vi "SW_Select_User_v.2.vi"() -> ()   [LabVIEW 2016]
uses:
  <vilib>/Utility/miscctls.llb/LVPointTypeDef.ctl
  <vilib>/Utility/config.llb/NI_LVConfig.lvlib
panel:
  out "TestComm indicator for Latching inside Events workaround":bool
  in  "Login tab":enum32{"Login", "Settings", "Manage users"}(tab)
  in  "Go to Tracker":bool
  in  "Select User":u16(ring) items=["Admin"]
  in  "Enter password":string
  in  "Jump to tracking":bool
  out "Comm. test results":bool
  in  "Test VISA Comms":bool
  in  "Save Settings":bool
  in  "VISA":refnum<visa-resource-name>="Tracker"
  in  "Cancel Users Update":bool
  in  "Save Users":bool
  in  "... or add new one":string
  in  "Reset or create password":string
  in  "Select User for update":u16(ring) items=["Researcher"]
  in  "Delete current user":bool
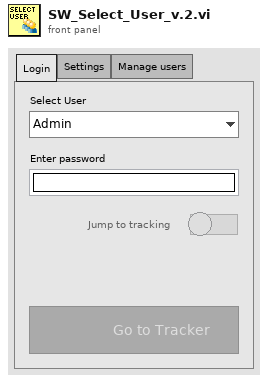
[diagram p1: front panel]
types:
  T1 = cluster{"Numeric Control":u32, "Numeric Control":u32}[]
  T2 = typedef "LVPointTypeDef.ctl" = cluster{"Horizontal":i16, "Vertical":i16}
  T3 = cluster{"Tabs":refnum<vi>, "Select User at login page":refnum<vi>, "Enter password":refnum<vi>, "Jump to tracking":refnum<vi>, "Test VISA Comms button":refnum<vi>, "Comm. test results indicator":refnum<vi>}
  T4 = typedef "NI_LVConfig.lvlib/Config Data RefNum.ctl" = refnum<k1>
  T5 = typedef "eventvkey.ctl" = enum16{"ASCII", "Enter", "Return", "Shift", "Ctrl", "Alt", "Cmd", "Opt", "Caps", "NumLock", "Clear", "Break", "Up", "Down", "Left", "Right", "Insert", "Delete", "Home", "End", "PageUp", "PageDown", "Escape", "Help", "Pause", "ScrollLock", "F1", "F2", "F3", "F4", "F5", "F6", "F7", "F8", "F9", "F10", "F11", "F12", "F13", "F14", "F15", "F16", "F17", "F18", "F19", "F20", "F21", "F22", "F23", "F24", "Play", "VolumeUp", "VolumeDown", "Mute", "Two Byte Char"}
  T6 = enum32{"Page Enabled", "Page Disabled", "Page Disabled & Grayed"}
  T7 = enum8{"Enabled", "Disabled", "Disabled and Grayed Out"}
  T8 = cluster{"Data acquisition status":refnum<notifier>, "Play/Pause status":refnum<notifier>, "Recording status":refnum<notifier>}
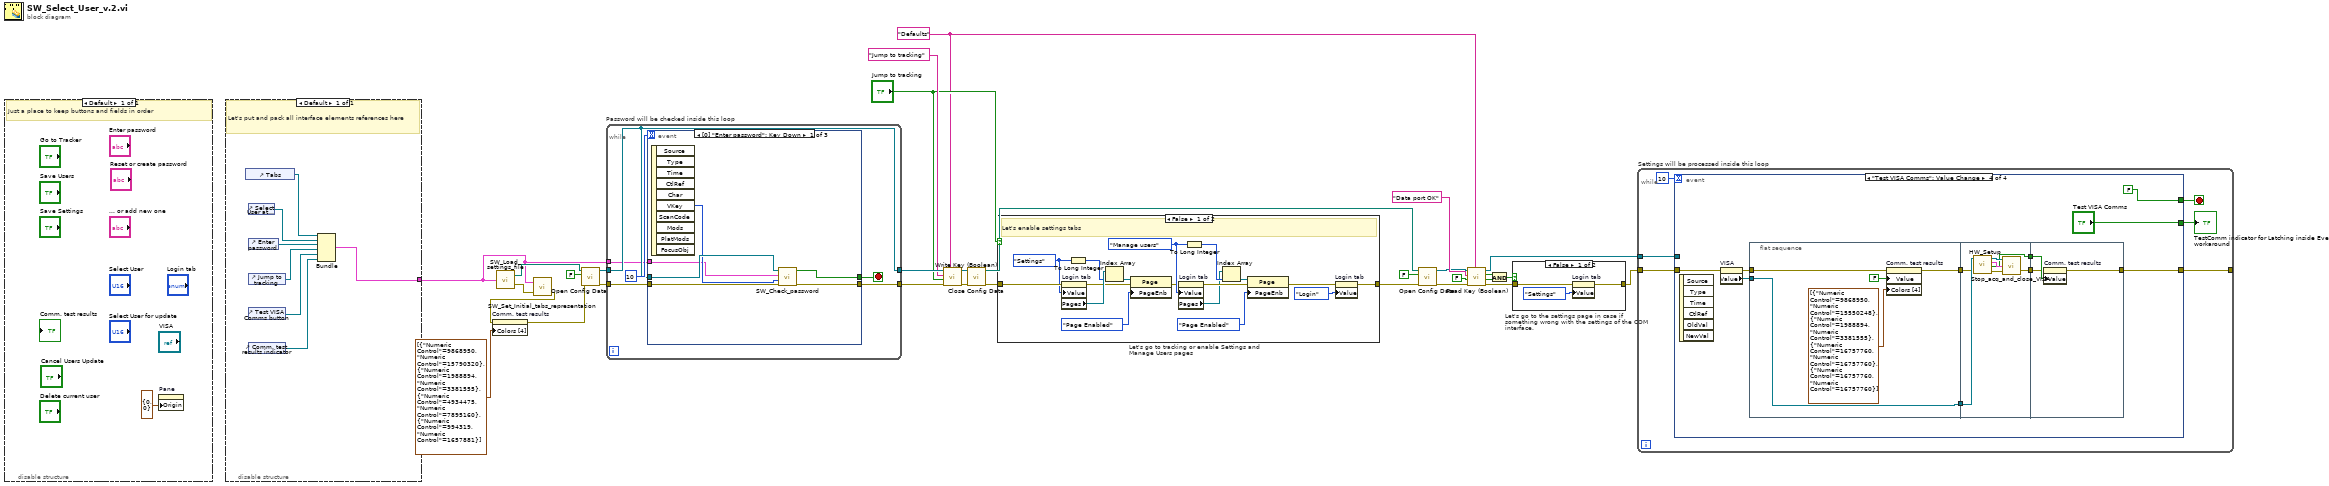
[diagram p0: block diagram]
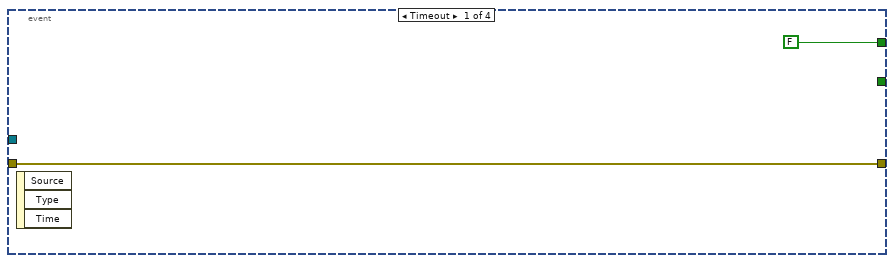
[diagram p2: hidden frame]
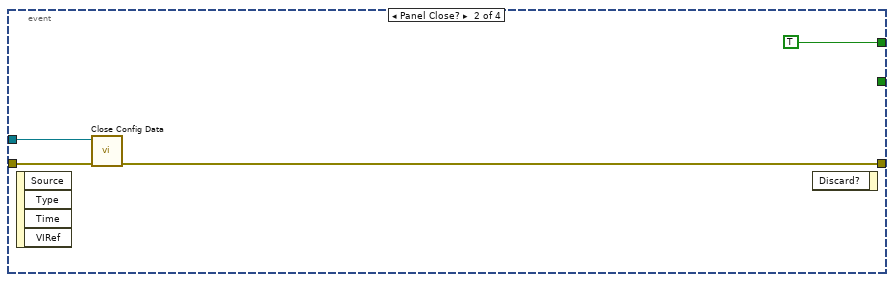
[diagram p3: hidden frame]
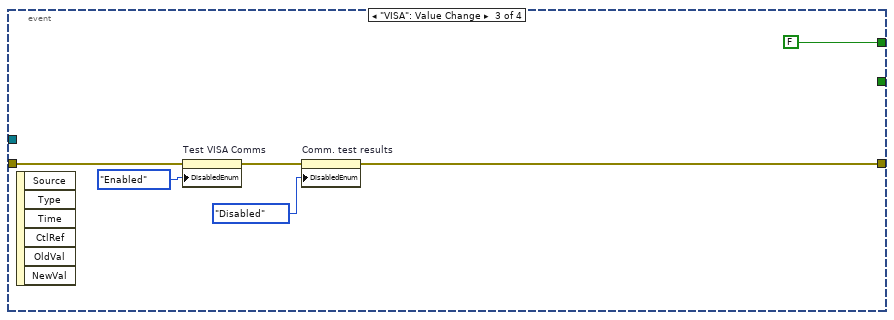
[diagram p4: hidden frame]
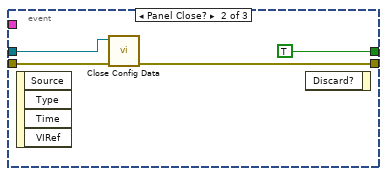
[diagram p7: hidden frame]
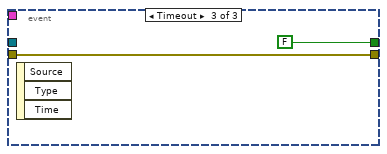
[diagram p8: hidden frame]
diagram:
  w22 = "Defaults" ("section")
  n1 = disable-structure shown="Default" {
    frame Enabled {
      # "Just a place to keep buttons and fields in order"
      n2 = property on="Pane" class="Pane"("Origin"=T2 {"Horizontal"=0, "Vertical"=0}) -> ()  [unwired: 2 in, 2 out]
    }
  }
  n3 = disable-structure "Conditional Disable Structure" shown="Default" {
    disable-tunnel: [w32] -> w1
    frame Enabled {
      # "Let's put and pack all interface elements references here"
      n4 = control-ref of="Tabs"() -> (w38:refnum<vi>)
      n5 = control-ref of="Select User at login page"() -> (w37:refnum<vi>)
      n6 = control-ref of="Enter password"() -> (w36:refnum<vi>)
      n7 = control-ref of="Jump to tracking"() -> (w35:refnum<vi>)
      n8 = control-ref of="Test VISA Comms button"() -> (w34:refnum<vi>)
      n9 = control-ref of="Comm. test results indicator"() -> (w33:refnum<vi>)
      n10 = Bundle("Tabs"=w38, "Select User at login page"=w37, "Enter password"=w36, "Jump to tracking"=w35, "Test VISA Comms button"=w34, "Comm. test results indicator"=w33) -> (w32:T3)  [unwired: 1 in]
    }
  }
  n11 = call "SW_Load_settings_file.vi"("Controls references"=w1) -> ("Config file path"=w7:path, "error out"=w28:errorcluster)
  n12 = call "SW_Set_Initial_tabs_representation.vi"("error in (no error)"=w28, "Controls references"=w1) -> ("error out"=w3:errorcluster)  [unwired: 1 in]
  n13 = property on="Comm. test results" class="Bool (strict)"(error in=w3, "Colors [4]"=T1 [{"Numeric Control"=9868950, "Numeric Control"=15790320}, {"Numeric Control"=1988894, "Numeric Control"=3381555}, {"Numeric Control"=4934475, "Numeric Control"=7895160}, {"Numeric Control"=994319, "Numeric Control"=1657881}]) -> (error out=w4:errorcluster)  [unwired: 1 in, 1 out]
  n14 = call <vilib>:"Open Config Data.vi"("error in (no error)"=w4, "create file if necessary (T)"=FALSE, "configuration file path"=w7) -> ("error out"=w29:errorcluster, "refnum"=w30:T4)  [unwired: 6 in, 1 out]
  n15 = while "Password will be checked inside this loop" {
    tunnel: w29 -> [w43]
    tunnel: w30 -> [w41]
    tunnel: [w42] -> w26
    tunnel: [w41] -> w27
    tunnel: w1 -> [w39]
    stop <- w40 stop-if-true
    n16 = event shown="[0] \"Enter password\": Key Down" {
      selector: _ -> [_ _ _]
      dyn-events: _ -> [_ _ _]
      timeout: 10 -> [_ _ _]
      tunnel: w43 -> [w50 w53 w55]
      tunnel: w41 -> [w49 w51 _]
      tunnel: [w47 TRUE ("Stop the loop") FALSE] -> w40
      tunnel: [w46 w52 w55] -> w42
      tunnel: w39 -> [w45 _ _]
      event "Enter password": Key Down {
        n17 = event-data() -> ("VKey"=w48:T5)  [unwired: 1 in, 9 out]
        n18 = call "SW_Check_password.vi"("error in (no error)"=w50, "Entered key"=w48, "Controls references"=w45, "Configuration file refnum in"=w49) -> ("error out"=w46:errorcluster, "Stop the loop"=w47:bool)  [unwired: 6 in]
      }
      event Panel Close? {
        n19 = event-data() -> ()  [unwired: 1 in, 4 out]
        n20 = call <vilib>:"Close Config Data.vi"("error in (no error)"=w53, "refnum"=w51) -> ("error out"=w52:errorcluster)  [unwired: 8 in, 1 out]
        n21 = event-data() -> ()  [unwired: 2 in, 1 out]
      }
      event Timeout {
        n22 = event-data() -> ()  [unwired: 1 in, 3 out]
      }
    }
  }
  n23 = call <vilib>:"Write Key (Boolean).vi"("section"=w22, "error in (no error)"=w26, "value"="Jump to tracking", "key"="Jump to tracking", "refnum"=w27) -> ("error out"=w16:errorcluster, "refnum out"=w14:T4)  [unwired: 4 in, 1 out]
  n24 = call <vilib>:"Close Config Data.vi"("error in (no error)"=w16, "refnum"=w14) -> ("error out"=w15:errorcluster, "file path"=w13:path)  [unwired: 8 in]
  n25 = case "Let's go to tracking or enable Settings and Manage Users pages" shown="False" "Jump to tracking" {
    tunnel: w15 -> [w73 w74]
    tunnel: [w58 w74] -> w12
    frame False {
      w62 = enum32{"Login", "Settings", "Manage users"}."Manage users" ("Login tab")
      w71 = enum32{"Login", "Settings", "Manage users"}."Settings" ("Login tab")
      # "Let's enable settings tabs"
      n26 = property on="Login tab" class="TabCtl (strict)"(error in=w73, "Value"=w71) -> (error out=w68:errorcluster, "Pages"=w72:refnum<vi>[])  [unwired: 1 in, 1 out]
      n27 = To Long Integer(number=w71) -> (32bit integer=w70:i32)
      n28 = Index Array(array=w72, index=w70) -> (element=w69:refnum<vi>)
      n29 = property class="Page"(reference=w69, error in=w68, "PageEnb"=T6."Page Enabled" ("Page Enabled State")) -> (error out=w60:errorcluster)  [unwired: 1 out]
      n30 = property on="Login tab" class="TabCtl (strict)"(error in=w60, "Value"=w62) -> (error out=w65:errorcluster, "Pages"=w61:refnum<vi>[])  [unwired: 1 in, 1 out]
      n31 = To Long Integer(number=w62) -> (32bit integer=w63:i32)
      n32 = Index Array(array=w61, index=w63) -> (element=w64:refnum<vi>)
      n33 = property class="Page"(reference=w64, error in=w65, "PageEnb"=T6."Page Enabled" ("Page Enabled State")) -> (error out=w59:errorcluster)  [unwired: 1 out]
      n34 = property on="Login tab" class="TabCtl (strict)"(error in=w59, "Value"=enum32{"Login", "Settings", "Manage users"}."Login" ("Login tab")) -> (error out=w58:errorcluster)  [unwired: 1 in, 1 out]
    }
    frame True {
      # "Here we'll check if everything else is OK and jump to tracking"
    }
  }
  n35 = call <vilib>:"Open Config Data.vi"("error in (no error)"=w12, "create file if necessary (T)"=FALSE, "configuration file path"=w13) -> ("error out"=w11:errorcluster, "refnum"=w10:T4)  [unwired: 6 in, 1 out]
  n36 = call <vilib>:"Read Key (Boolean).vi"("section"=w22, "error in (no error)"=w11, "default value"=FALSE, "key"="Data port OK", "refnum"=w10) -> ("error out"=w17:errorcluster, "value"=w19:bool, "found?"=w20:bool, "refnum out"=w5:T4)  [unwired: 3 in]
  n37 = And(x=w20, y=w19) -> (x .and. y?=w18:bool)
  n38 = case "Let's go to the settings page in case if something wrong with the settings of the COM interface." shown="False" w18 {
    tunnel: w17 -> [w75 w78]
    tunnel: [w77 w78] -> w6
    frame False {
      n39 = property on="Login tab" class="TabCtl (strict)"(error in=w75, "Value"=enum32{"Login", "Settings", "Manage users"}."Settings" ("Login tab")) -> (error out=w77:errorcluster)  [unwired: 1 in, 1 out]
    }
    frame True {
    }
  }
  n40 = while "Settings will be processed inside this loop" {
    tunnel: w6 -> [w82]
    tunnel: [w83] -> _
    tunnel: w5 -> [w80]
    stop <- w81 stop-if-true
    n41 = event shown="[3] \"Test VISA Comms\": Value Change" {
      selector: _ -> [_ _ _ _]
      dyn-events: _ -> [_ _ _ _]
      timeout: 10 -> [_ _ _ _]
      tunnel: [w86 w87 w92 w100] -> w83
      tunnel: w82 -> [w86 w88 w96 w105]
      tunnel: [FALSE TRUE FALSE FALSE] -> w81
      tunnel: w80 -> [_ w89 _ _]
      tunnel: [_ _ _ "Test VISA Comms"] -> w79
      event Timeout {
        n42 = event-data() -> ()  [unwired: 1 in, 3 out]
      }
      event Panel Close? {
        n43 = event-data() -> ()  [unwired: 1 in, 4 out]
        n44 = call <vilib>:"Close Config Data.vi"("error in (no error)"=w88, "refnum"=w89) -> ("error out"=w87:errorcluster)  [unwired: 8 in, 1 out]
        n45 = event-data() -> ()  [unwired: 2 in, 1 out]
      }
      event "VISA": Value Change {
        n46 = event-data() -> ()  [unwired: 1 in, 6 out]
        n47 = property on="Test VISA Comms" class="Bool"(error in=w96, "DisabledEnum"=T7."Enabled" ("Disabled")) -> (error out=w95:errorcluster)  [unwired: 1 in, 1 out]
        n48 = property on="Comm. test results" class="Bool (strict)"(error in=w95, "DisabledEnum"=T7."Disabled" ("Disabled")) -> (error out=w92:errorcluster)  [unwired: 1 in, 1 out]
      }
      event "Test VISA Comms": Value Change {
        n49 = event-data() -> ()  [unwired: 1 in, 6 out]
        n50 = property on="VISA" class="VISAName"(error in=w105) -> (error out=w104:errorcluster, "Value"=w103:refnum<visa-resource-name>)  [unwired: 1 in, 1 out]
        n51 = flat-sequence {
          tunnel: w104 -> [w109]
          tunnel: w103 -> [w111]
          tunnel: [w111] -> w102
          tunnel: [w108] -> w101
          tunnel: w102 -> [w118]
          tunnel: w101 -> [w113]
          tunnel: [w114] -> w98
          tunnel: [w112] -> w97
          tunnel: [w121] -> w100
          tunnel: w97 -> [w119]
          tunnel: w98 -> [w120]
          frame #0 {
            n52 = property on="Comm. test results" class="Bool (strict)"(error in=w109, "Value"=FALSE ("Comm. test results"), "Colors [4]"=T1 [{"Numeric Control"=9868950, "Numeric Control"=15550248}, {"Numeric Control"=1988894, "Numeric Control"=3381555}, {"Numeric Control"=16757760, "Numeric Control"=16757760}, {"Numeric Control"=16757760, "Numeric Control"=16757760}]) -> (error out=w108:errorcluster)  [unwired: 1 in, 1 out]
          }
          frame #1 {
            n53 = call "HW_Setup.vi"("VISA resource name in"=w118, "error in"=w113) -> ("VISA resource name out"=w117:refnum<visa-resource-name>, "Data flow controls"=w116:T8, "Instrument OK?"=w114:bool, "error out"=w115:errorcluster)  [unwired: 1 in]
            n54 = call "Stop_acq_and_close_VISA.vi"("error in"=w115, "Data flow controls in"=w116, "VISA resource name in"=w117) -> ("error out"=w112:errorcluster)  [unwired: 1 out]
          }
          frame #2 {
            n55 = property on="Comm. test results" class="Bool (strict)"(error in=w119, "Value"=w120) -> (error out=w121:errorcluster)  [unwired: 1 in, 1 out]
          }
        }
      }
    }
    "TestComm indicator for Latching inside Events workaround" <- w79
  }
